vi "Write_parameter.vi"(8 "error in (no error)":errorcluster caption="entrée d'erreur (pas d'erreur)", 10 "Parameter":string, 11 "Class Instrument (Default) en entrée":refnum<class "Class Instrument Printer.lvclass">) -> (0 "error out":errorcluster caption="sortie d'erreur", 3 "Class Instrument (Default) en sortie":refnum<class "Class Instrument Printer.lvclass">)   [LabVIEW 2020, in "Library Instrument & Equipement.lvlib" / "Library Instruments.lvlib" / "Class Instrument Printer.lvclass"]
uses:
  Class Instrument Printer.lvclass
  Commun VI/TypeDef/Commande Printer/Commande Parameter Printer.ctl
  Printer/Printer (Default)/Class Printer (Default).lvclass
  Class Instrument Printer.lvclass/Class Instrument Printer.ctl
  JSON API/JSON Value/Set from JSON string.vi
  Instrument (Default)/Class Instrument (Default).lvclass
  JSON API/JSON Value/JSON Value.lvclass
  JSON API/Variant JSON/Variant JSON.lvlib
  JSON API/Get Polymorphic/JSON GetSet.lvlib
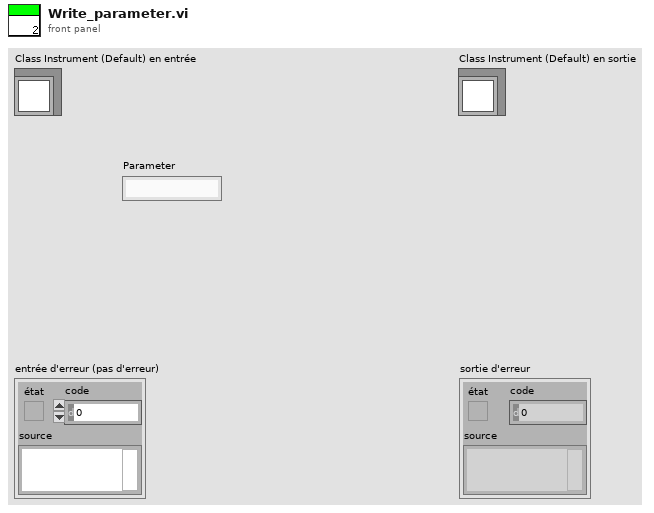
[diagram p1: front panel]
types:
  T1 = typedef "Commande Parameter Printer.ctl" = cluster{"Device_Printer":string, "File To print":path, "Path Picture":path, "Library Printer":refnum<class "Class Printer (Default).lvclass">}
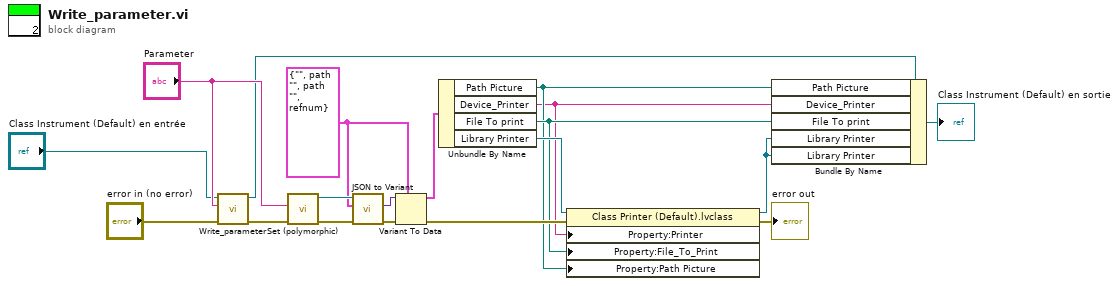
[diagram p0: block diagram]
diagram:
  w14 = T1 {"Device_Printer"="", "File To print"=path "", "Path Picture"=path "", "Library Printer"=refnum} ("Parameter")
  n1 = call-parent "Write_parameter.vi"("error in (no error)"="error in (no error)", "Parameter"="Parameter", "Class Instrument (Default) en entrée"="Class Instrument (Default) en entrée") -> ("error out"=w15:errorcluster, "Class Instrument (Default) en sortie"=w8:refnum<class "Class Instrument Printer.lvclass">)  [unwired: 7 in]
  n2 = call-poly "Set (polymorphic).vi"("error in (no error)"=w15, "JSON stream"="Parameter") -> ("error out"=w17:errorcluster, "JSON Value out"=w19:refnum<class "JSON Value.lvclass">)  [unwired: 7 in, 1 out]
  n3 = call "JSON to Variant.vi"("error in (no error)"=w17, "Variant (Data Type)"=w14, "JSON Value"=w19) -> ("error out"=w18:errorcluster, "Variant out"=w16:variant)  [unwired: 7 in]
  n4 = Variant To Data(error in=w18, type=w14, Variant=w16) -> (data=w12:T1, error out=w6:errorcluster)
  n5 = Unbundle By Name(w12) -> ("Path Picture"=w2:path, "Device_Printer"=w1:string, "File To print"=w3:path, "Library Printer"=w7:refnum<class "Class Printer (Default).lvclass">)
  n6 = property class="Class Printer (Default).lvclass"(reference=w7, error in=w6, "Property:Printer"=w1, "Property:File_To_Print"=w3, "Property:Path Picture"=w2) -> (reference out=w4:refnum<class "Class Printer (Default).lvclass">, error out=→"error out":errorcluster)
  n7 = Bundle By Name(cluster=w8, "Path Picture"=w2, "Device_Printer"=w1, "File To print"=w3, "Library Printer"=w4, "Library Printer"=w4) -> (→"Class Instrument (Default) en sortie":refnum<class "Class Instrument Printer.lvclass">)
